vi "Net_Probe.vi"(11 "NET":refnum<class "NET.lvclass">) -> (2 "Value String":string, 3 "Pause VI":bool)   [LabVIEW 2020, in "OpenLvVision_OpenCv.lvlib" / "NET.lvclass"]
uses:
  NET.lvclass
  C:/Users/lukas/Downloads/OpenLvVision_OpenCv/SourceCode/LabView/OpenLvVision_OpenCv/_LvHelpers/EdvrObject/EdvrObject.lvclass
  _LvHelpers/EdvrObject/EdvrObject.lvclass/EdvrObject.ctl
  _LvHelpers/EdvrObject/EdvrObject.lvclass
panel:
  out "LayerNames":string[](array[string])
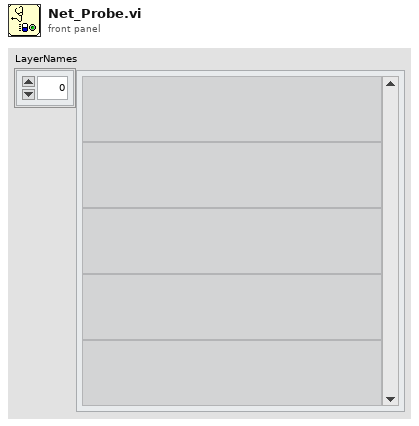
[diagram p1: front panel]
types:
  T1 = typedef "OpenLvVision_OpenCv.lvlib/EdvrObject.lvclass/Edvr.ctl" = refnum<data-value>
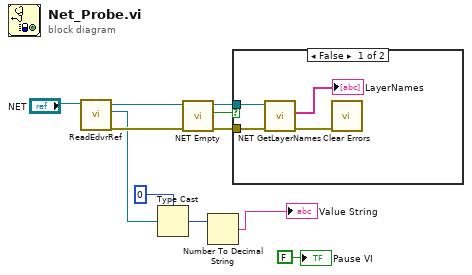
[diagram p0: block diagram]
diagram:
  n1 = call "ReadEdvrRef.vi"("EdvrObject in"="NET") -> ("error out"=w5:errorcluster, "Edvr"=w4:T1, "EdvrObject out"=w6:refnum<class "NET.lvclass">)  [unwired: 8 in]
  n2 = Type Cast(type=0, x=w4) -> (*(type *) &x=w2:i32)
  n3 = call "NET Empty.vi"("error in (no error)"=w5, "NET in"=w6) -> ("error out"=w8:errorcluster, "Emtpy"=w10:bool, "NET out"=w9:refnum<class "NET.lvclass">)  [unwired: 7 in]
  n4 = Number To Decimal String(number=w2) -> (decimal integer string=→"Value String":string)  [unwired: 1 in]
  n5 = case shown="False" w10 {
    tunnel: w9 -> [w15 _]
    tunnel: w8 -> [w14 _]
    frame False {
      n6 = call "NET GetLayerNames.vi"("error in (no error)"=w14, "NET in"=w15) -> ("error out"=w12:errorcluster, "LayerNames"=→"LayerNames":string[])  [unwired: 7 in, 1 out]
      n7 = call <vilib>:"Clear Errors.vi"("error in (no error)"=w12) -> ()  [unwired: 5 in, 2 out]
    }
    frame True {
    }
  }
  "Pause VI" <- FALSE
